vi "Arduino Output.vi"() -> ()   [LabVIEW 2013, in "LVH-LINX.lvlib"]
doc: "Read one the value of one analog channel from a LINX device."
uses:
  <vilib>/LabVIEW Hacker/LINX/LVH-LINX.lvlib
  <vilib>/LabVIEW Hacker/LINX/Public/Peripherals/Analog/Analog Read 1 Chan.vi
  C:/Users/Beads/Downloads/Agilis Labview drivers 7.1/Agilis Labview 7.1/AGILIS.llb/enter / leave remote mode.vi
panel:
  in  "SerialPort (1)":u8=1
  out "Timeout":bool
  in  "Jog":i32(knob) min=-3 max=3 scale=-3.0..3.0
  in  "stop 2":bool
  in  "Axis":u32=1
  out "stop":bool
  in  "AI Channel":u8
  out "Loop Rate (Hz)":u32
  in  "Stop Button":bool
  out "Analog Data":dbl(graph)
  in  "Serial Port":refnum<visa-resource-name>
  # "Voltage, A0"
  # "LINX Device Settings"
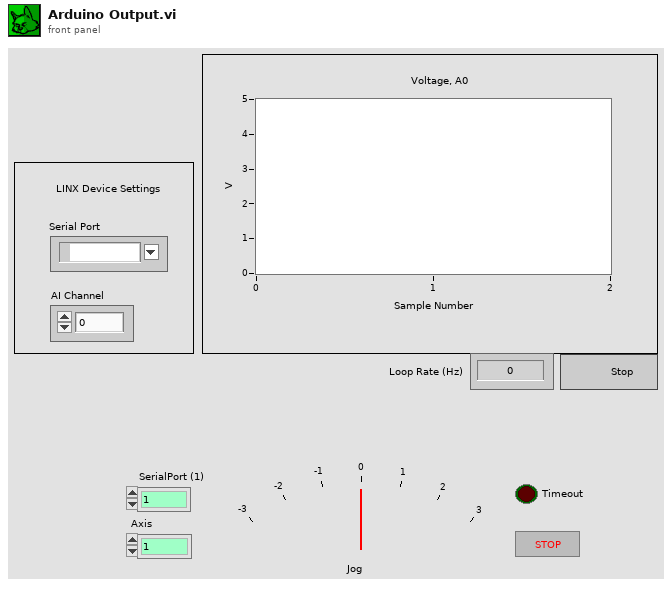
[diagram p1: front panel]
types:
  T1 = typedef "LVH-LINX.lvlib/LINX Ref.ctl" = cluster{"Platform":T2, "Interface":T3, "LINX Device Config":T4}
  T2 = typedef "LVH-LINX.lvlib/Platform.ctl" = enum16{"LINX", "myRIO"}
  T3 = typedef "LVH-LINX.lvlib/Interface.ctl" = enum16{"Serial", "TCP"}
  T4 = typedef "LVH-LINX.lvlib/Device.lvlib/LINX Device Config.ctl" = cluster{"Interface":T3, "COM Port":refnum<visa-resource-name>, "TCP Configuration":T5, "Device Family":T6, "Device ID":u8, "Device Name":string, "TCP Ref":refnum<k5>}
  T5 = typedef "LVH-LINX.lvlib/Device.lvlib/TCP Config.ctl" = cluster{"IP Address":string, "Port":u16}
  T6 = typedef "LVH-LINX.lvlib/Device Family.ctl" = enum8{"National Instruments", "Digilent", "Arduino"}
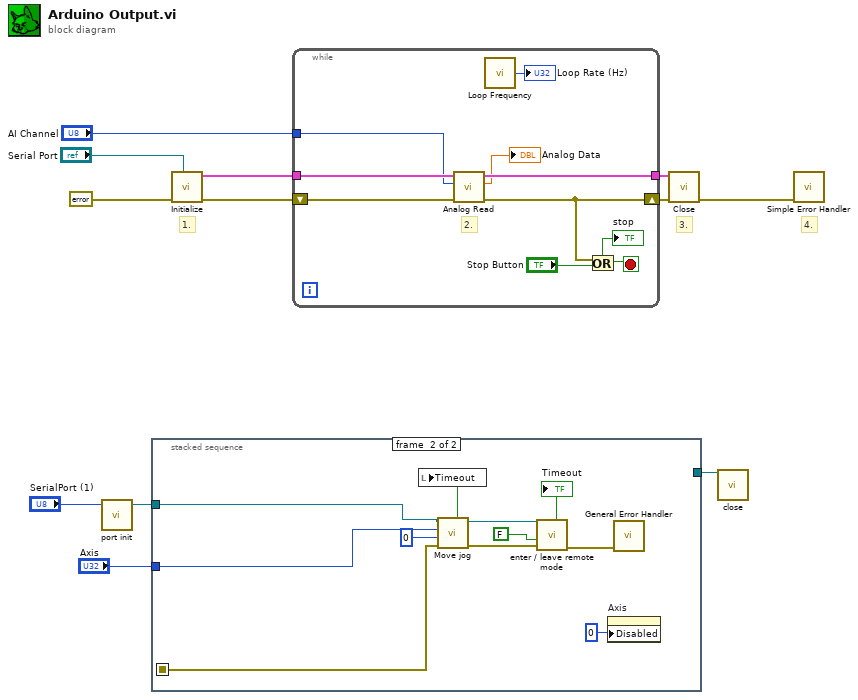
[diagram p0: block diagram]
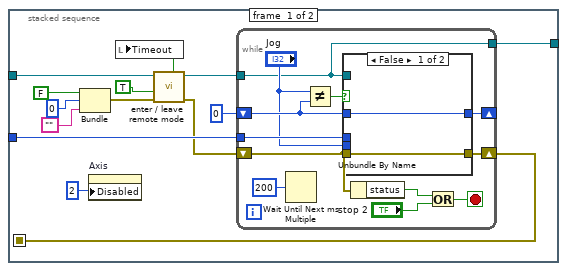
[diagram p2: hidden frame]
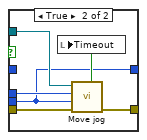
[diagram p3: hidden frame]
diagram:
  # "4."
  # "3."
  # "1."
  n1 = call "port init.vi"("SerialPort (1)"="SerialPort (1)") -> ("Visa Handle"=w3:refnum<visa-resource-name>)  [unwired: 3 in, 1 out]
  n2 = stacked-sequence {
    seq-local: [w24 _] -> [_ w55]
    tunnel: w3 -> [w17 w48]
    tunnel: "Axis" -> [w26 w57]
    tunnel: [w13 _] -> w1
    frame #0 {
      n3 = Bundle(FALSE, 0, "") -> (w19:errorcluster)  [unwired: 1 in]
      n4 = property on="Axis" class="DigNum (strict)"("Disabled"=u8 2 ("Désactivé")) -> ()  [unwired: 2 in, 2 out]
      n5 = call "enter / leave remote mode.vi"("error in"=w19, "enter / disable remote mode (True)"=TRUE, "VISA handle in"=w17) -> ("error out"=w15:errorcluster, "VISA handle out"=w16:refnum<visa-resource-name>, "TimeoutFlag"=w18:bool)  [unwired: 6 in]
      n6 = local write "Timeout"(w18) -> ()
      n7 = while {
        tunnel: w16 -> [w27]
        tunnel: w26 -> [w38]
        shift-right: [w36] -> _
        shift-left: 0 -> [w30]
        shift-right: [w35] -> w24
        shift-left: w15 -> [w34]
        tunnel: [w27] -> w13
        stop <- w32 stop-if-true
        n8 = Wait Until Next ms Multiple(millisecond multiple=u32 200 ("n millisecondes")) -> ()  [unwired: 1 out]
        n9 = Not Equal?(x="Jog", y=w30) -> (x != y?=w37:bool)
        n10 = case shown="False" w37 {
          tunnel: w34 -> [w39 w46]
          tunnel: w27 -> [_ w44]
          tunnel: w38 -> [_ w43]
          tunnel: "Jog" -> [_ w42]
          tunnel: [w40 w42] -> w36
          tunnel: w30 -> [w40 _]
          tunnel: [w39 w41] -> w35
          frame False {
          }
          frame True {
            n11 = call <userlib>:"Move jog.vi"("error in"=w46, "Jog mode"=w42, "Axis in"=w43, "VISA Handle in"=w44) -> ("error out"=w41:errorcluster, "TimeoutFlag"=w45:bool)  [unwired: 2 in, 2 out]
            n12 = local write "Timeout"(w45) -> ()
          }
        }
        n13 = Unbundle By Name(w34) -> ("status"=w31:bool)
        n14 = Or(x=w31, y="stop 2") -> (x .or. y?=w32:bool)
      }
    }
    frame #1 {
      n15 = call <userlib>:"Move jog.vi"("error in"=w55, "Jog mode"=0, "Axis in"=w57, "VISA Handle in"=w48) -> ("error out"=w53:errorcluster, "VISA Handle out"=w54:refnum<visa-resource-name>, "TimeoutFlag"=w50:bool)  [unwired: 2 in, 1 out]
      n16 = local write "Timeout"(w50) -> ()
      n17 = call "enter / leave remote mode.vi"("error in"=w53, "enter / disable remote mode (True)"=FALSE, "VISA handle in"=w54) -> ("error out"=w47:errorcluster, "TimeoutFlag"=→"Timeout":bool)  [unwired: 6 in, 1 out]
      n18 = property on="Axis" class="DigNum (strict)"("Disabled"=u8 0 ("Désactivé")) -> ()  [unwired: 2 in, 2 out]
      n19 = call <vilib>:"General Error Handler.vi"("error in (no error)"=w47) -> ()  [unwired: 10 in, 5 out]
    }
  }
  n20 = call <vilib>:"Initialize.vi"("Serial Port"="Serial Port", "Error In"=errorcluster {"status"=FALSE, "code"=0, "source"=""}) -> ("Error Out"=w11:errorcluster, "LINX Ref"=w12:T1)  [unwired: 7 in, 1 out]
  n21 = while {
    tunnel: w12 -> [w66]
    tunnel: [w64] -> w10
    shift-right: [w61] -> w9
    shift-left: w11 -> [w65]
    tunnel: "AI Channel" -> [w59]
    stop <- w63 stop-if-true
    # "2."
    n22 = call-poly <vilib>:"Analog Read.vi"("Error In"=w65, "Analog Channel"=w59, "LINX Resource"=w66) -> ("Error Out"=w61:errorcluster, "AI Value"=→"Analog Data":dbl, "LINX Resource"=w64:T1)  [unwired: 5 in, 1 out]
    n23 = call <vilib>:"Loop Frequency.vi"() -> ("Loop Rate (Hz)"=→"Loop Rate (Hz)":u32)
    n24 = Or(x=w61, y="Stop Button") -> (x .or. y?=w63:bool)
    "stop" <- w63
  }
  n25 = call <vilib>:"Close.vi"("Error In"=w9, "LINX Resource"=w10) -> ("Error Out"=w7:errorcluster)  [unwired: 8 in, 1 out]
  n26 = call <vilib>:"close.vi"("VISA Handle in"=w1) -> ()  [unwired: 4 in, 1 out]
  n27 = call <vilib>:"Simple Error Handler.vi"("error in (no error)"=w7) -> ()  [unwired: 4 in, 5 out]
